vi "sub_trigger-check2.vi"(8 "error in (no error)":errorcluster caption="에러 입력(에러 없음)", 11 "wf in":waveform(dbl)) -> (0 "error out":errorcluster caption="에러 출력", 3 "stop trigger":bool)   [LabVIEW 2013]
uses:
  <vilib>/measure/mamon.llb/Trigger Detection for 1 Channel.vi
  <vilib>/measure/NI_MAPro.lvlib
panel:
  out "웨이브폼 그래프":waveform(dbl)(graph)
  out "x > y?":bool
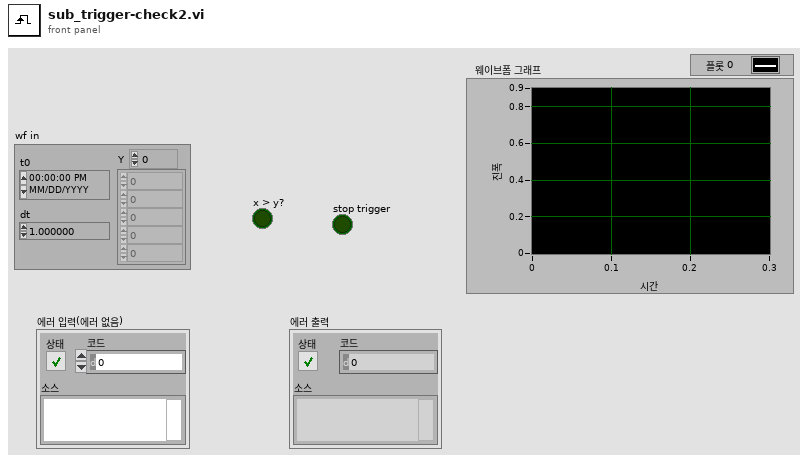
[diagram p1: front panel]
types:
  T1 = typedef "config_ctl.ctl" = cluster{"Trigger minlevel":dbl, "Lower Cut-Off":dbl, "Force high_level":dbl, "state settings":cluster{"method":enum32{"histogram", "peak", "auto select"}, "histogram size":i32, "histogram method":enum16{"mode"}, "reserved":dbl}}
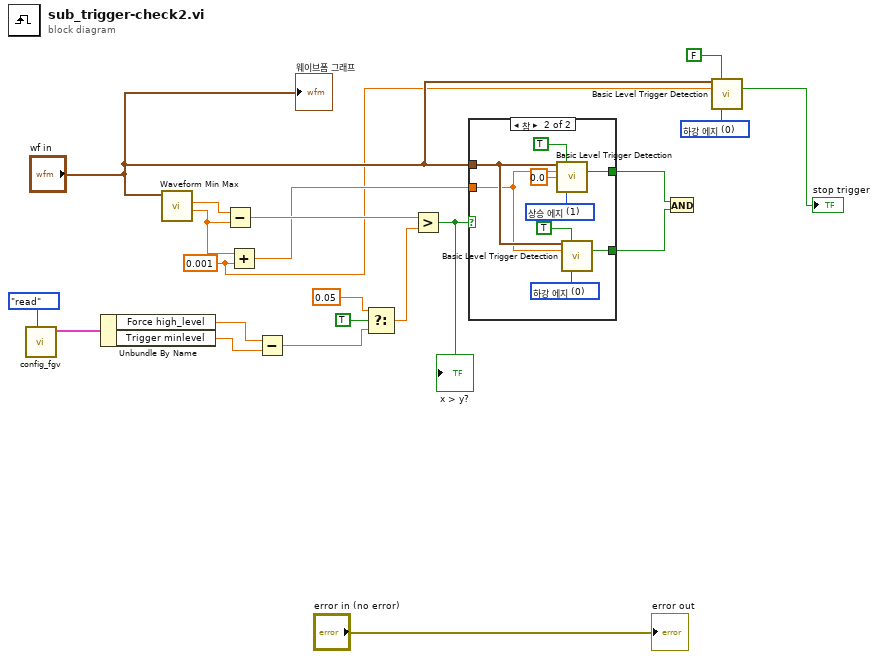
[diagram p0: block diagram]
diagram:
  w5 = u16 0 items=["하강 에지", "상승 에지"] ("trigger slope")
  w1 = 0.001 ("y")
  n1 = call "config_fgv.vi"("cmd"=enum16{"write", "read", "ini"}."read") -> ("Config out"=w20:T1)  [unwired: 9 in, 1 out]
  n2 = Unbundle By Name(w20) -> ("Force high_level"=w16:dbl, "Trigger minlevel"=w15:dbl)
  n3 = call <vilib>:"Waveform Min Max.vi"("waveform in"="wf in") -> ("Y min"=w7:dbl, "Y max"=w18:dbl)  [unwired: 5 in, 4 out]
  n4 = Subtract(x=w18, y=w7) -> (x-y=w17:dbl)
  n5 = Add(x=w7, y=w1) -> (x+y=w6:dbl)
  n6 = Subtract(x=w16, y=w15) -> (x-y=w11:dbl)
  n7 = Select(t=0.05, s=TRUE, f=w11) -> (s? t:f=w8:dbl)
  n8 = Greater?(x=w17, y=w8) -> (0:w14:bool)
  "x > y?" <- w14
  n9 = case shown="참" w14 {
    tunnel: "wf in" -> [_ w28]
    tunnel: [_ w27] -> w13
    tunnel: [_ w26] -> w12
    tunnel: w6 -> [_ w25]
    frame False {
    }
    frame True {
      w29 = u16 0 items=["하강 에지", "상승 에지"] ("trigger slope")
      w30 = u16 1 items=["하강 에지", "상승 에지"] ("trigger slope")
      n10 = call-poly <vilib>:"Basic Level Trigger Detection.vi"("signal in"=w28, "reset"=TRUE, "level"=w25, "hysteresis"=0.0, "trigger slope"=w30) -> ("trigger detected?"=w26:bool)  [unwired: 8 in, 2 out]
      n11 = call-poly <vilib>:"Basic Level Trigger Detection.vi"("signal in"=w28, "reset"=TRUE, "level"=w25, "trigger slope"=w29) -> ("trigger detected?"=w27:bool)  [unwired: 9 in, 2 out]
    }
  }
  n12 = And(x=w12, y=w13) -> ()  [unwired: 1 out]
  n13 = call-poly <vilib>:"Basic Level Trigger Detection.vi"("signal in"="wf in", "reset"=FALSE, "level"=w1, "trigger slope"=w5) -> ("trigger detected?"=→"stop trigger":bool)  [unwired: 9 in, 2 out]
  "error out" <- "error in (no error)"
  "웨이브폼 그래프" <- "wf in"
